vi "MathOptim-Sigmoid Invert.vi"(7 "Parameters":dbl[](array[numeric]), 11 "Y":dbl format="%.2f") -> (8 "X":dbl)   [LabVIEW 2020]
doc: "This template is the starting point for creating a model function to be passed to the Nonlinear Curve Fit.vi."
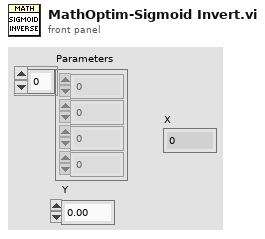
[diagram p1: front panel]
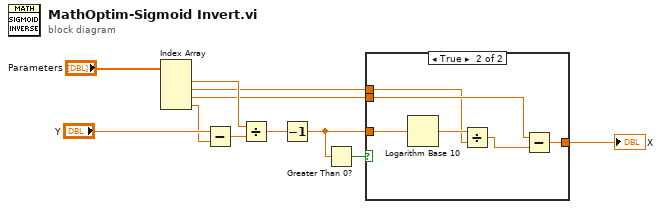
[diagram p0: block diagram]
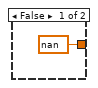
[diagram p2: hidden frame]
diagram:
  n1 = Index Array(array="Parameters") -> (element #1=w7:dbl, element #2=w3:dbl, element #3=w4:dbl, element #4=w8:dbl)  [unwired: 4 in]
  n2 = Subtract(x="Y", y=w8) -> (x-y=w9:dbl)
  n3 = Divide(x=w7, y=w9) -> (x/y=w6:dbl)
  n4 = Decrement(x=w6) -> (x-1=w5:dbl)
  n5 = Greater Than 0?(x=w5) -> (x > 0?=w1:bool)
  n6 = case shown="True" w1 {
    tunnel: w5 -> [_ w17]
    tunnel: w4 -> [_ w18]
    tunnel: w3 -> [_ w15]
    tunnel: [nan w13] -> w2
    frame False {
    }
    frame True {
      n7 = Logarithm Base 10(1:w17) -> (0:w16:dbl)
      n8 = Divide(x=w16, y=w15) -> (x/y=w14:dbl)
      n9 = Subtract(x=w18, y=w14) -> (x-y=w13:dbl)
    }
  }
  "X" <- w2
